vi "Full Trace Log.vi"(8 "error in (no error)":errorcluster, 11 "RequestTraceLog in":refnum<class "RequestTraceLog.lvclass">) -> (0 "error out":errorcluster, 2 "Trace Log":T1 {"Sending" format="%_6f"; "Expires" format="%<%X %x>T"; "Created" format="%<%X %x>T"; "Waiting" format="%_6f"; "Parsing" format="%_6f"; "Processing" format="%_6f"; "Items"."Time" format="%.6f"; "Items"."Duration" format="%.6f"}, 3 "RequestTraceLog out":refnum<class "RequestTraceLog.lvclass">)   [LabVIEW 2020, in "HTTP Server.lvlib" / "RequestTraceLog.lvclass"]
uses:
  RequestTraceLog.lvclass
  Trace Log.ctl
  Trace Item.ctl
  Processing Step.ctl
  lv-http-util/HTTP Utils/Method.ctl
  RequestTraceLog.lvclass/RequestTraceLog.ctl
  HTTP Server.lvlib
  lv-http-util/HTTP Utils/HTTP Utils.lvlib
  lv-uri/URI/URI/URI.lvclass
panel:
  # "Request"
  # "Response"
  # "Session"
  # "Auth"
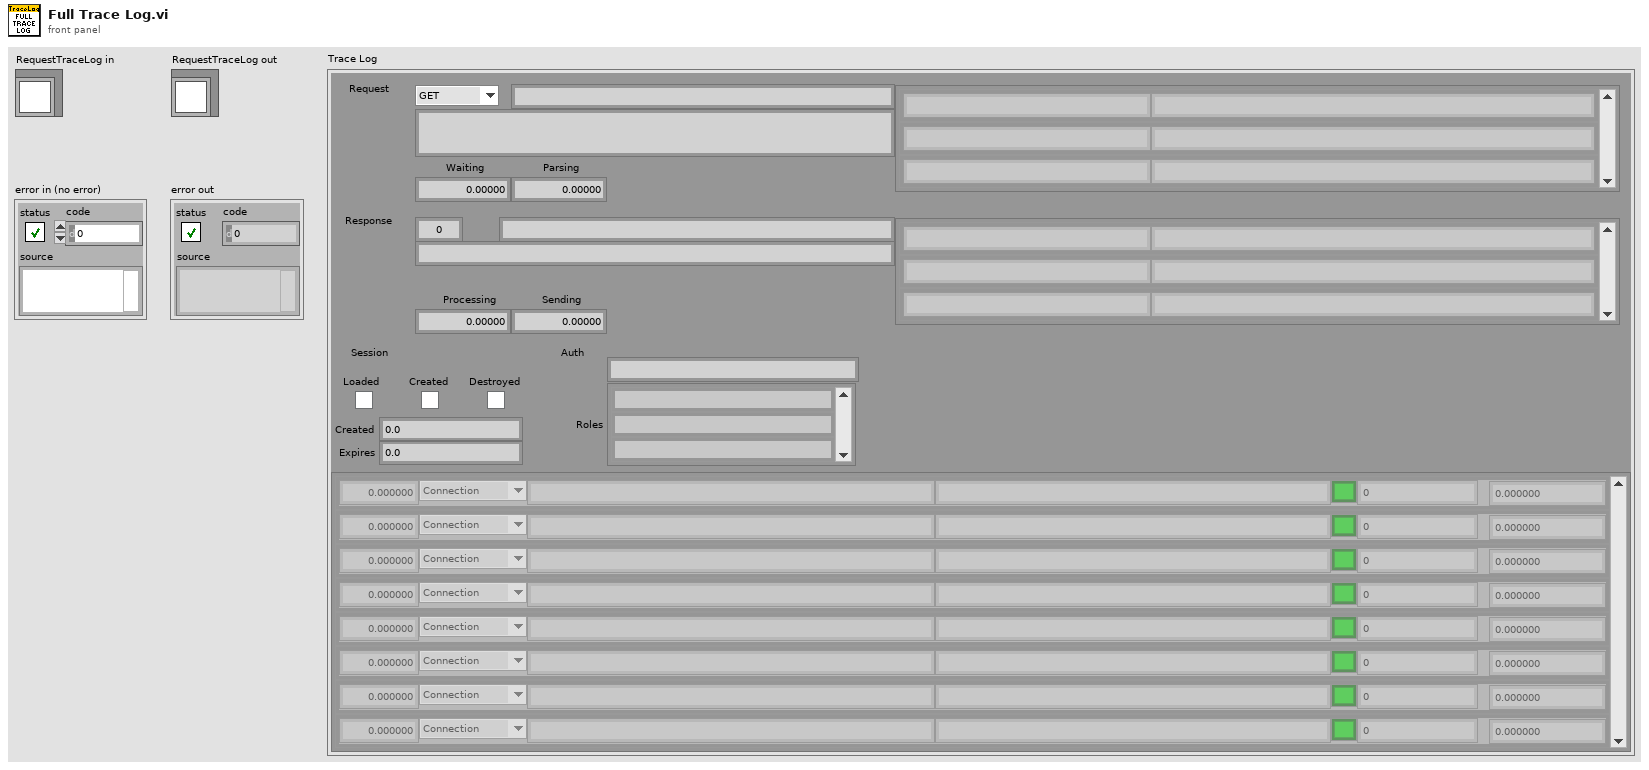
[diagram p1: front panel]
types:
  T1 = typedef "HTTP Server.lvlib/Trace Log.ctl" = cluster{"Items":T2[], "Client":string, "Target":string, "Response Type":string, "Processing":dbl, "Status":u16, "Method":T4, "Content Type":string, "Request Headers":cluster{"Name":string, "Value":string}[], "Parsing":dbl, "Waiting":dbl, "Identity":string, "Loaded":bool, "Created":bool, "Destroyed":bool, "Response Headers":cluster{"Name":string, "Value":string}[], "Created":dbl, "Expires":dbl, "Roles":string[], "Sending":dbl}
  T2 = typedef "HTTP Server.lvlib/Trace Item.ctl" = cluster{"Duration":dbl, "Step":T3, "Class":string, "Info":string, "Status":bool, "Code":i32, "Time":dbl}
  T3 = typedef "HTTP Server.lvlib/Processing Step.ctl" = enum16{"Connection", "Request", "Routing", "Controller Init", "Controller", "Response", "Complete", "Exception"}
  T4 = typedef "HTTP Utils.lvlib/Method.ctl" = enum16{"GET", "HEAD", "POST", "PUT", "DELETE", "CONNECT", "OPTIONS", "TRACE", "PATCH"}
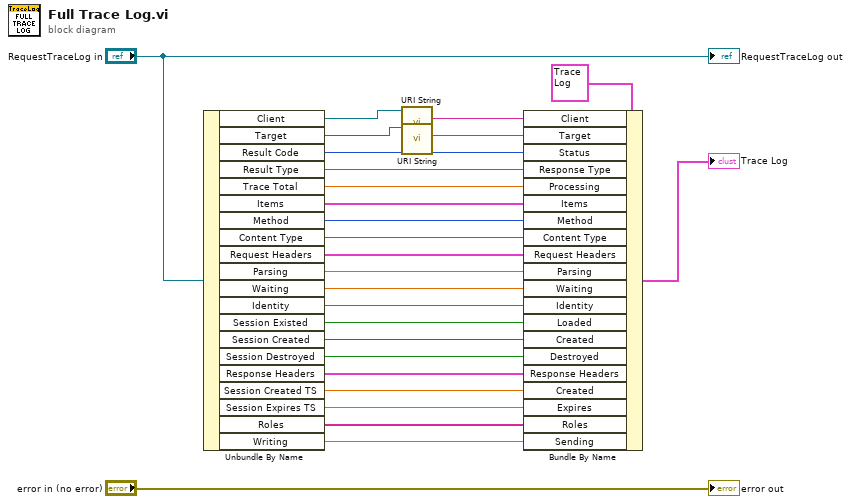
[diagram p0: block diagram]
diagram:
  n1 = Unbundle By Name("RequestTraceLog in") -> ("Client"=w16:refnum<class "URI.lvclass">, "Target"=w18:refnum<class "URI.lvclass">, "Result Code"=w22:u16, "Result Type"=w21:string, "Trace Total"=w20:dbl, "Items"=w19:T2[], "Method"=w14:T4, "Content Type"=w13:string, "Request Headers"=w12:cluster{"Name":string, "Value":string}[], "Parsing"=w11:dbl, "Waiting"=w10:dbl, "Identity"=w9:string, "Session Existed"=w8:bool, "Session Created"=w7:bool, "Session Destroyed"=w6:bool, "Response Headers"=w5:cluster{"Name":string, "Value":string}[], "Session Created TS"=w4:dbl, "Session Expires TS"=w3:dbl, "Roles"=w2:string[], "Writing"=w1:dbl)
  n2 = call "URI String.vi"("URI in"=w16) -> ("URI String"=w15:string)  [unwired: 9 in, 1 out]
  n3 = call "URI String.vi"("URI in"=w18) -> ("URI String"=w17:string)  [unwired: 9 in, 1 out]
  n4 = Bundle By Name(cluster=T1 {"Items"=[], "Client"="", "Target"="", "Response Type"="", "Processing"=0.0, "Status"=0, "Method"=enum."GET", "Content Type"="", "Request Headers"=[], "Parsing"=0.0, "Waiting"=0.0, "Identity"="", "Loaded"=FALSE, "Created"=FALSE, "Destroyed"=FALSE, "Response Headers"=[], "Created"=0.0, "Expires"=0.0, "Roles"=[], "Sending"=0.0} ("Trace Log"), "Client"=w15, "Target"=w17, "Status"=w22, "Response Type"=w21, "Processing"=w20, "Items"=w19, "Method"=w14, "Content Type"=w13, "Request Headers"=w12, "Parsing"=w11, "Waiting"=w10, "Identity"=w9, "Loaded"=w8, "Created"=w7, "Destroyed"=w6, "Response Headers"=w5, "Created"=w4, "Expires"=w3, "Roles"=w2, "Sending"=w1) -> (→"Trace Log":T1)
  "error out" <- "error in (no error)"
  "RequestTraceLog out" <- "RequestTraceLog in"
